vi "DT_Merge_Two Subsets.vi"(5 "right subset":i32, 7 "left subset":i32, 9 "Subset Triangles In":cluster{"Triangles":i32[][]}[](array[cluster]), 10 "Subset":cluster{"start idx":i32, "length":i32}[](array[cluster]), 11 "Points In":cluster{"x":dbl, "y":dbl, "index":i32}[](array[cluster])) -> (0 "error":i32, 1 "Subset Triangles Out":cluster{"Triangles":i32[][]}[](array[cluster]), 3 "Points Out":cluster{"x":dbl, "y":dbl, "index":i32}[](array[cluster]))   [LabVIEW 2017, in "NI_AAL_Geometry.lvlib"]
uses:
  <vilib>/Analysis/NI_AAL_Geometry.lvlib
  <vilib>/Analysis/geometry.llb/DT_Cal Length.vi
  <vilib>/Analysis/baseanly.llb/Determinant.vi
  <vilib>/Analysis/baseanly.llb/Real Determinant.vi
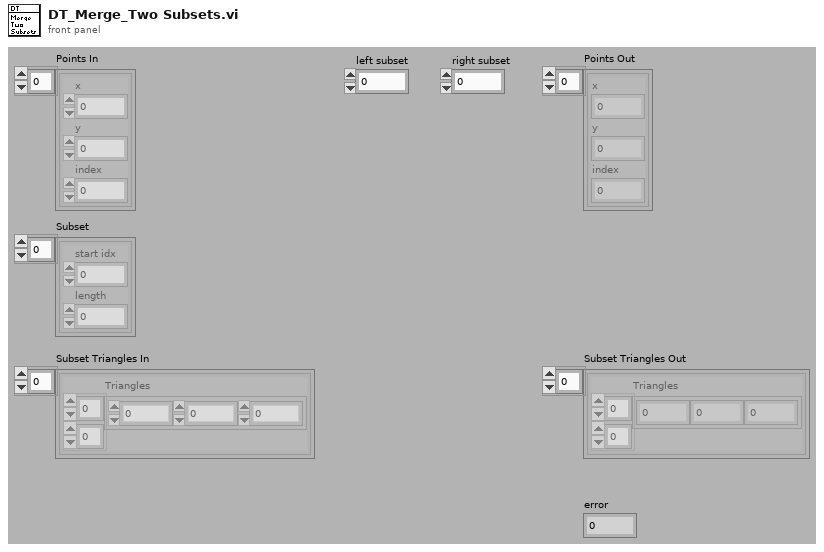
[diagram p1: front panel]
types:
  T1 = typedef "NI_AAL_Geometry.lvlib/DT_Merge_Find Next Triangulation_Data.ctl" = cluster{"left base point":i32, "left triangle":i32, "left local idx":i32, "right base point":i32, "right triangle":i32, "right local idx":i32, "Left Candidate Triangles":i32[], "Left Candidate Point Idx":i32[], "Right Candidate Triangles":i32[], "Right Candidate Point Idx":i32[], "cur triangle":i32}
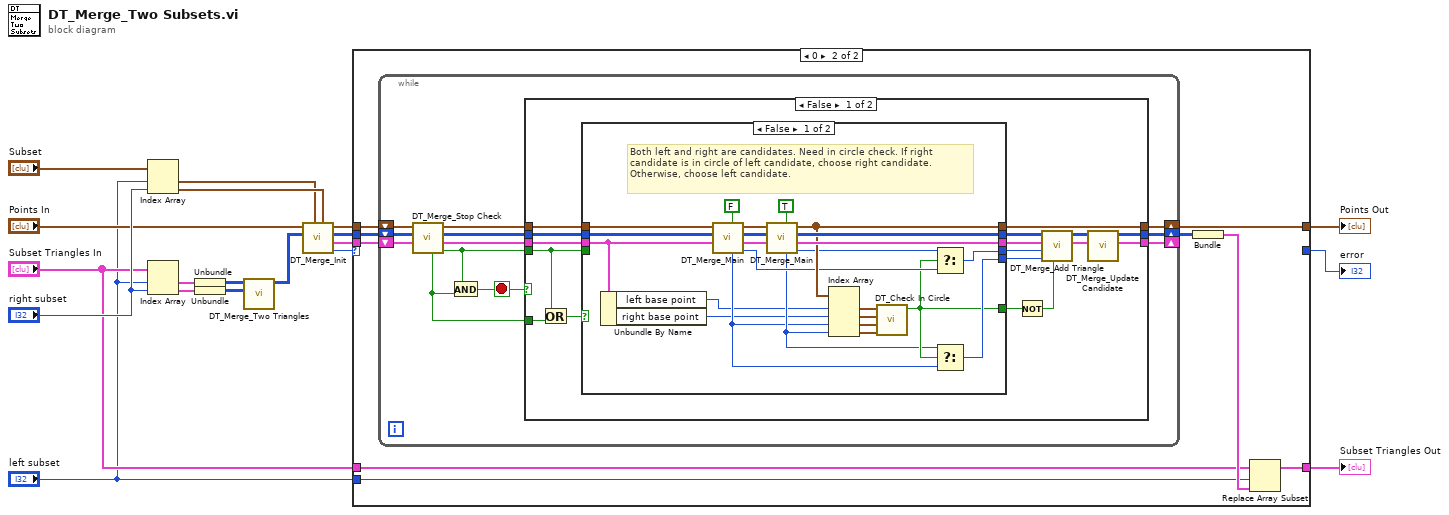
[diagram p0: block diagram]
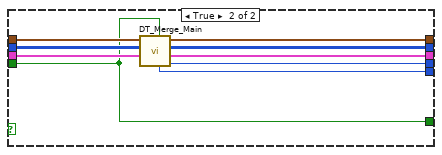
[diagram p3: hidden frame]
diagram:
  n1 = Index Array(array="Subset", index #1="left subset", index #2="right subset") -> (element #1=w5:cluster{"start idx":i32, "length":i32}, element #2=w13:cluster{"start idx":i32, "length":i32})
  n2 = Index Array(array="Subset Triangles In", index #1="left subset", index #2="right subset") -> (element #1=w18:cluster{"Triangles":i32[][]}, element #2=w17:cluster{"Triangles":i32[][]})
  n3 = Unbundle(w18) -> ("Triangles"=w15:i32[][])
  n4 = Unbundle(w17) -> ("Triangles"=w14:i32[][])
  n5 = call <vilib>:"DT_Merge_Two Triangles.vi"("Right Triangles"=w14, "Left Triangles"=w15) -> ("Merged Triangles"=w12:i32[][])  [unwired: 2 in, 7 out]
  n6 = call <vilib>:"DT_Merge_Init.vi"("right subset"=w13, "left subset"=w5, "Triangles In"=w12, "Points In"="Points In") -> ("error"=w2:i32, "Data"=w7:T1, "Triangles Out"=w8:i32[][], "Points Out"=w9:cluster{"x":dbl, "y":dbl, "index":i32}[])  [unwired: 4 out]
  n7 = case shown="0" w2 {
    selector: w2 -> [w20 _]
    tunnel: [_ w28] -> w10
    tunnel: w9 -> [_ w27]
    tunnel: w8 -> [_ w26]
    tunnel: w7 -> [_ w25]
    tunnel: [_ w23] -> w6
    tunnel: "Subset Triangles In" -> [_ w22]
    tunnel: "left subset" -> [_ w21]
    tunnel: [w20 _] -> w1
    frame Default {
    }
    frame 0 {
      n8 = while {
        shift-right: [w32] -> w23
        shift-left: w27 -> [w41]
        shift-right: [w31] -> w24
        shift-left: w26 -> [w40]
        shift-right: [w30] -> _
        shift-left: w25 -> [w39]
        stop <- w38 stop-if-true
        n9 = call <vilib>:"DT_Merge_Stop Check.vi"("Data In"=w39, "Triangles In"=w40, "Points In"=w41) -> ("left stop?"=w34:bool, "Data Out"=w37:T1, "Triangles Out"=w36:i32[][], "Points Out"=w35:cluster{"x":dbl, "y":dbl, "index":i32}[], "right stop?"=w33:bool)  [unwired: 4 out]
        n10 = And(x=w34, y=w33) -> (x .and. y?=w38:bool)
        n11 = case shown="False" w38 {
          tunnel: w37 -> [w56 w92]
          tunnel: w36 -> [w57 w93]
          tunnel: w35 -> [w58 w94]
          tunnel: w34 -> [w53 _]
          tunnel: w33 -> [w54 _]
          tunnel: [w46 w94] -> w32
          tunnel: [w43 w93] -> w31
          tunnel: [w42 w92] -> w30
          frame False {
            n12 = Or(x=w53, y=w54) -> (x .or. y?=w55:bool)
            n13 = case shown="False" w55 {
              tunnel: w58 -> [w82 w91]
              tunnel: w57 -> [w81 w90]
              tunnel: w56 -> [w73 w84]
              tunnel: w53 -> [_ w83]
              tunnel: [w72 w89] -> w46
              tunnel: [w75 w88] -> w51
              tunnel: [w74 w87] -> w50
              tunnel: [w65 w86] -> w49
              tunnel: [w64 w85] -> w48
              tunnel: [w63 w83] -> w52
              frame False {
                # "Both left and right are candidates. Need in circle check. If right candidate is in circle of left candidate, choose right candidate. Otherwise, choose left candidate."
                n14 = Unbundle By Name(w73) -> ("left base point"=w59:i32, "right base point"=w60:i32)
                n15 = call <vilib>:"DT_Merge_Main.vi"("left/right pt (right:F)"=FALSE, "Data In"=w73, "Triangles In"=w81, "Points In"=w82) -> ("triangle"=w66:i32, "Data Out"=w78:T1, "Triangles Out"=w79:i32[][], "Points Out"=w80:cluster{"x":dbl, "y":dbl, "index":i32}[], "point"=w61:i32)  [unwired: 1 in, 2 out]
                n16 = call <vilib>:"DT_Merge_Main.vi"("left/right pt (right:F)"=TRUE, "Data In"=w78, "Triangles In"=w79, "Points In"=w80) -> ("triangle"=w67:i32, "Data Out"=w74:T1, "Triangles Out"=w75:i32[][], "Points Out"=w72:cluster{"x":dbl, "y":dbl, "index":i32}[], "point"=w62:i32)  [unwired: 1 in, 2 out]
                n17 = Index Array(array=w72, index #1=w59, index #2=w60, index #3=w61, index #4=w62) -> (element #1=w71:cluster{"x":dbl, "y":dbl, "index":i32}, element #2=w70:cluster{"x":dbl, "y":dbl, "index":i32}, element #3=w69:cluster{"x":dbl, "y":dbl, "index":i32}, element #4=w68:cluster{"x":dbl, "y":dbl, "index":i32})
                n18 = call <vilib>:"DT_Check In Circle.vi"("p 4"=w68, "p 3"=w69, "p 2"=w70, "p 1"=w71) -> ("in circle?"=w63:bool)  [unwired: 7 out]
                n19 = Select(t=w67, s=w63, f=w66) -> (s? t:f=w65:i32)
                n20 = Select(t=w62, s=w63, f=w61) -> (s? t:f=w64:i32)
              }
              frame True {
                n21 = call <vilib>:"DT_Merge_Main.vi"("left/right pt (right:F)"=w83, "Data In"=w84, "Triangles In"=w90, "Points In"=w91) -> ("triangle"=w86:i32, "Data Out"=w87:T1, "Triangles Out"=w88:i32[][], "Points Out"=w89:cluster{"x":dbl, "y":dbl, "index":i32}[], "point"=w85:i32)  [unwired: 1 in, 2 out]
              }
            }
            n22 = Not(x=w52) -> (.not. x?=w47:bool)
            n23 = call <vilib>:"DT_Merge_Add Triangle.vi"("left/right pt (right:F)"=w47, "point"=w48, "triangle"=w49, "Data In"=w50, "Triangles In"=w51) -> ("Data Out"=w44:T1, "Triangles Out"=w45:i32[][])  [unwired: 5 out]
            n24 = call <vilib>:"DT_Merge_Update Candidate.vi"("Data In"=w44, "Triangles In"=w45) -> ("Data Out"=w42:T1, "Triangles Out"=w43:i32[][])  [unwired: 1 in, 7 out]
          }
          frame True {
          }
        }
      }
      n25 = Bundle("Triangles Out"=w24) -> (w29:cluster{"Triangles Out":i32[][]})  [unwired: 1 in]
      n26 = Replace Array Subset(array=w22, new element=w29, index=w21) -> (w28:cluster{"Triangles":i32[][]}[])
    }
  }
  "Points Out" <- w6
  "Subset Triangles Out" <- w10
  "error" <- w1
